vi "APS pt spiral ca.vi"(7 "Status":T1, 8 "error in (no error)":errorcluster caption="错误输入（无错误）", 9 "Prof":cluster{"Angle":dbl, "DeltaH":dbl, "FinalR":dbl}, 10 "PtbId":i32, 11 "Board_ID":i32) -> (0 "error out":errorcluster caption="错误输出", 1 "Prof out":cluster{"Angle":dbl, "DeltaH":dbl, "FinalR":dbl}, 3 "function return":i32, 5 "Status out":T1)   [LabVIEW 2011, in "APS168.lvlib"]
doc: "I32 FNTYPE APS_pt_spiral_ca( I32 Board_ID, I32 PtbId, PPTHCA Prof, PPTSTS Status );"
uses:
  APS168.lvlib
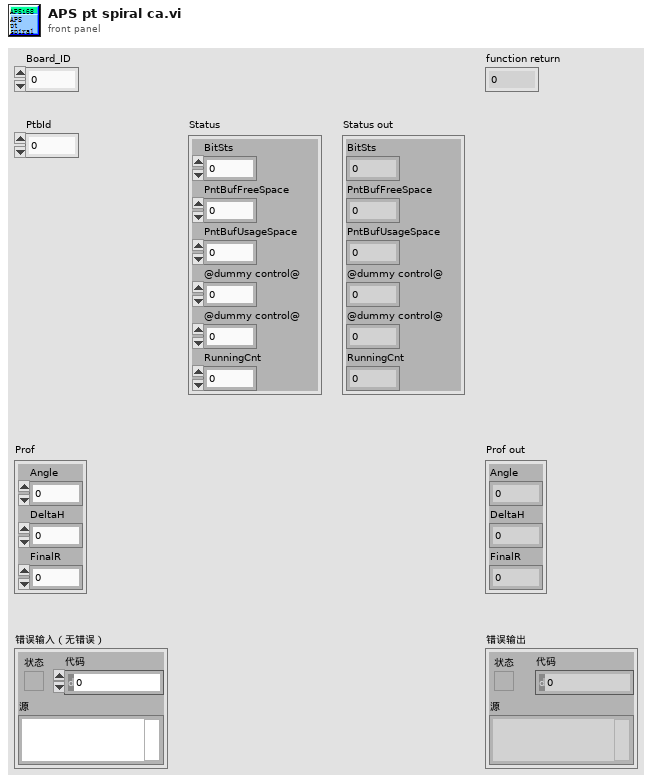
[diagram p1: front panel]
types:
  T1 = cluster{"BitSts":u16, "PntBufFreeSpace":u16, "PntBufUsageSpace":u16, "@dummy control@":i8, "@dummy control@":i8, "RunningCnt":u32}
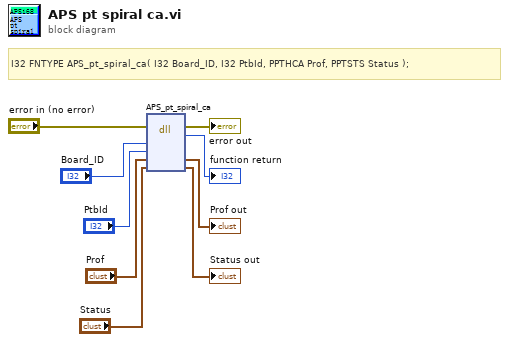
[diagram p0: block diagram]
diagram:
  # "I32 FNTYPE APS_pt_spiral_ca( I32 Board_ID, I32 PtbId, PPTHCA Prof, PPTSTS Status );"
  n1 = dll-call lib="PTH1Labs E软件ADLINK 204CAPS_1_7_1_LIB line 连续运动204APS168.*" fn="APS_pt_spiral_ca"(error in="error in (no error)", "Board_ID"="Board_ID", "PtbId"="PtbId", "Prof"="Prof", "Status"="Status") -> (error out=→"error out":errorcluster, →"function return":i32, "Prof"=→"Prof out":cluster{"Angle":dbl, "DeltaH":dbl, "FinalR":dbl}, "Status"=→"Status out":T1)  [unwired: 4 in, 1 out]
